vi "Trim Ends.vi"(1 "String":string) -> (0 "Trimmed String":string)   [LabVIEW 2012, in "OPI.lvclass"]
uses:
  OPI.lvclass
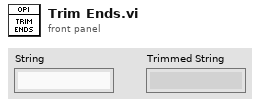
[diagram p1: front panel]
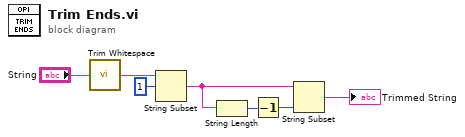
[diagram p0: block diagram]
diagram:
  n1 = call <vilib>:"Trim Whitespace.vi"("string"="String") -> ("trimmed string"=w1:string)  [unwired: 1 in]
  n2 = String Subset(string=w1, offset (0)=1) -> (substring=w7:string)  [unwired: 1 in]
  n3 = String Length(string=w7) -> (length=w5:i32)
  n4 = Decrement(x=w5) -> (x-1=w6:i32)
  n5 = String Subset(string=w7, length (rest)=w6) -> (substring=→"Trimmed String":string)  [unwired: 1 in]
